vi "Import Pictures from Files.vi"(0 "Display State In":T1, 7 "Pictures":path[](array[path]), 9 "Container State":T3, 11 "error in (no error)":errorcluster) -> (4 "Display State Out":T1, 15 "error out":errorcluster)   [LabVIEW 2016]
uses:
  <vilib>/Utility/miscctls.llb/LVBoundsTypeDef.ctl
  HorizontalList.xctl
  <vilib>/_xctls/Container State.ctl
  <vilib>/_xctls/XControlSupport.lvlib
  HorizontalList_State.ctl
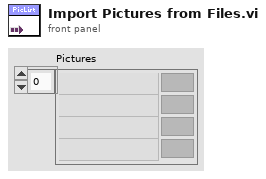
[diagram p1: front panel]
types:
  T1 = typedef "HorizontalList.xctl/HorizontalList_State.ctl" = cluster{"Persistent":cluster{"Elements":string[], "PicElements":picture[], "Limits":i32[], "Selection":picture[], "Selection Color":u32, "Highlight":picture[], "Highlight Val":i32, "Highlight Color":u32}, "Draw Area Size":T2, "List Ref":refnum<vi>, "Visible":u8}
  T2 = typedef "LVBoundsTypeDef.ctl" = cluster{"Width":u32, "Height":u32}
  T3 = typedef "XControlSupport.lvlib/Container State.ctl" = cluster{"Indicator?":bool, "Run Mode?":bool, " Refnum":refnum<vi>}
  T4 = typedef "imagedata.ctl" = cluster{"image type":i32, "image depth":i32, "image":u8[], "mask":u8[], "colors":u32[], "Rectangle":cluster{"left":i16, "top":i16, "right":i16, "bottom":i16}}
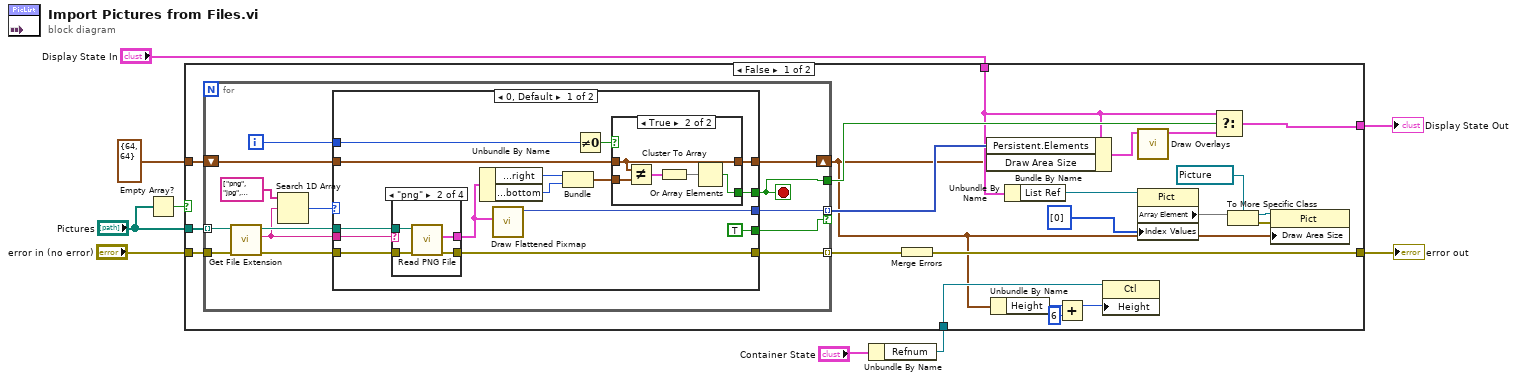
[diagram p0: block diagram]
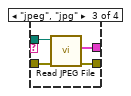
[diagram p4: hidden frame]
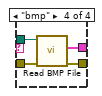
[diagram p5: hidden frame]
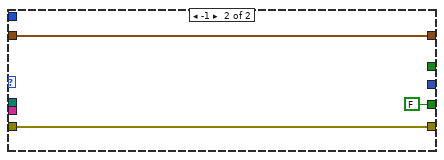
[diagram p6: hidden frame]
diagram:
  n1 = Empty Array?(array="Pictures") -> (empty?=w4:bool)
  n2 = Unbundle By Name("Container State") -> ("Refnum"=w1:refnum<vi>)
  n3 = case shown="False" w4 {
    tunnel: "Pictures" -> [w31 _]
    tunnel: "error in (no error)" -> [w30 w84]
    tunnel: [w27 w84] -> w8
    tunnel: T2 {"Width"=64, "Height"=64} ("Draw Area Size") -> [w26 _]
    tunnel: [w24 w83] -> w6
    tunnel: "Display State In" -> [w23 w83]
    tunnel: w1 -> [w14 _]
    frame False {
      n4 = for {
        tunnel: w31 -> [w45] mode=indexing
        tunnel: w30 -> [w43]
        tunnel: [w41] -> w29 mode=indexing if=w32
        tunnel: [w40] -> w28 mode=indexing
        shift-right: [w37] -> w13
        shift-left: w26 -> [w38]
        tunnel: [w36] -> w25
        i -> [w39]
        stop <- w36 stop-if-true
        n5 = call <vilib>:"Get File Extension.vi"("error in (no error)"=w43, "file"=w45) -> ("error out"=w42:errorcluster, "lowercase file extension"=w34:string, "dup file"=w44:path)  [unwired: 5 in, 2 out]
        n6 = Search 1D Array(1D array=string[] ["png", "jpg", "jpeg", "bmp"], element=w34) -> (index of element=w33:i32)  [unwired: 1 in]
        n7 = case shown="0, Default" w33 {
          tunnel: w44 -> [w60 _]
          tunnel: w42 -> [w59 w81]
          tunnel: [w58 _] -> w41
          tunnel: [w57 w81] -> w40
          tunnel: w39 -> [w55 _]
          tunnel: w38 -> [w51 w82]
          tunnel: [w50 w82] -> w37
          tunnel: [w48 _] -> w36
          tunnel: w34 -> [w47 _]
          tunnel: [TRUE FALSE] -> w32
          frame 0, Default {
            n8 = case shown="\"png\"" w47 {
              tunnel: w60 -> [_ w71 w75 w79]
              tunnel: w59 -> [w67 w70 w74 w78]
              tunnel: [_ w69 w72 w76] -> w56
              tunnel: [w67 w68 w73 w77] -> w57
              frame Default {
              }
              frame "png" {
                n9 = call <vilib>:"Read PNG File.vi"("error in (no error)"=w70, "path to PNG file"=w71) -> ("error out"=w68:errorcluster, "image data"=w69:T4)  [unwired: 7 in, 1 out]
              }
              frame "jpeg", "jpg" {
                n10 = call <vilib>:"Read JPEG File.vi"("error in (no error)"=w74, "path to JPEG file"=w75) -> ("error out"=w73:errorcluster, "image data"=w72:T4)  [unwired: 7 in, 1 out]
              }
              frame "bmp" {
                n11 = call <vilib>:"Read BMP File.vi"("error in (no error)"=w78, "path to BMP file"=w79) -> ("error out"=w77:errorcluster, "image data"=w76:T4)  [unwired: 7 in, 1 out]
              }
            }
            n12 = Unbundle By Name(w56) -> ("Rectangle.right"=w54:i16, "Rectangle.bottom"=w53:i16)
            n13 = call <vilib>:"Draw Flattened Pixmap.vi"("image data"=w56) -> ("new picture"=w58:picture)  [unwired: 8 in]
            n14 = Bundle("right"=w54, "bottom"=w53) -> (w49:cluster{"right":i16, "bottom":i16})  [unwired: 1 in]
            n15 = Not Equal To 0?(x=w55) -> (x != 0?=w52:bool)
            n16 = case shown="True" w52 {
              tunnel: w51 -> [_ w66]
              tunnel: [w61 w66] -> w50
              tunnel: w49 -> [w61 w65]
              tunnel: [_ w62] -> w48
              frame False {
              }
              frame True {
                n17 = Not Equal?(x=w66, y=w65) -> (x != y?=w64:cluster{bool, bool})
                n18 = Cluster To Array(cluster=w64) -> (array=w63:bool[])
                n19 = Or Array Elements(Boolean array=w63) -> (logical OR=w62:bool)
              }
            }
          }
          frame -1 {
          }
        }
      }
      n20 = Merge Errors(w28) -> (w27:errorcluster)
      n21 = Bundle By Name(cluster=w23, "Persistent.Elements"=w29, "Draw Area Size"=w13) -> (w11:T1)
      n22 = Unbundle By Name(w13) -> ("Height"=w17:u32)
      n23 = Unbundle By Name(w23) -> ("List Ref"=w22:refnum<vi>)
      n24 = Add(x=w17, y=u32 6) -> (x+y=w16:u32)
      n25 = property class="Ctl"(reference=w14, "Height"=w16) -> ()  [unwired: 1 in, 2 out]
      n26 = call "Draw Overlays.vi"("Default Control State in"=w11) -> ("Default Control State out"=w10:T1)  [unwired: 10 in]
      n27 = property class="Pict"(reference=w22, "Index Values"=u32[] [0]) -> ("Array Element"=w21)  [unwired: 1 in, 2 out]
      n28 = Select(t=w23, s=w25, f=w10) -> (s? t:f=w24:T1)
      n29 = To More Specific Class(target class=refnum<vi> refnum ("reference"), reference=w21) -> (specific class reference=w19:refnum<vi>, error out=w18:errorcluster)  [unwired: 1 in]
      n30 = property class="Pict"(reference=w19, error in=w18, "Draw Area Size"=w13) -> ()  [unwired: 2 out]
    }
    frame True {
    }
  }
  "Display State Out" <- w6
  "error out" <- w8
